vi "Temperature.vi"(7 "SlaveID":u8=1, 8 "error in (no error)":errorcluster, 11 ".NET Refnum in":refnum<k24>) -> (0 "error out":errorcluster, 2 "Temperature":dbl, 3 "reference out":refnum<k24>)   [LabVIEW 2017]
uses:
  DLL/Modbus.dll
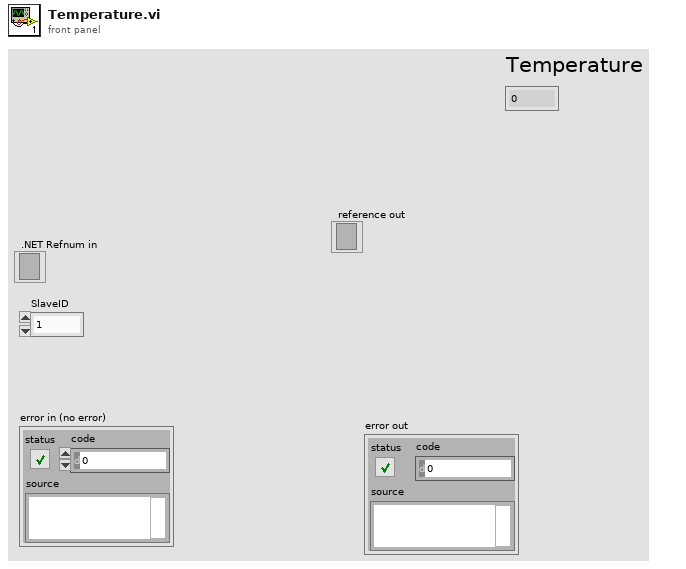
[diagram p1: front panel]
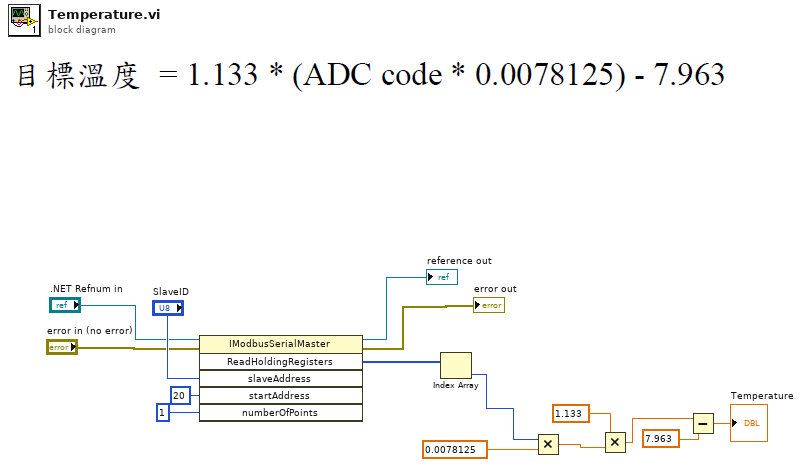
[diagram p0: block diagram]
diagram:
  n1 = invoke class="IModbusSerialMaster" method="ReadHoldingRegisters"(reference=".NET Refnum in", error in="error in (no error)", "slaveAddress"="SlaveID", "startAddress"=u16 20, "numberOfPoints"=u16 1) -> (reference out=→"reference out":refnum<k24>, error out=→"error out":errorcluster, "ReadHoldingRegisters"=w10:u16[])  [unwired: 1 in, 3 out]
  n2 = Index Array(array=w10) -> (element=w2:u16)  [unwired: 1 in]
  n3 = Multiply(x=w2, y=0.0078125) -> (x*y=w6:dbl)
  n4 = Multiply(x=1.133, y=w6) -> (x*y=w4:dbl)
  n5 = Subtract(x=w4, y=7.963) -> (x-y=→"Temperature":dbl)
